vi "Teleop.vi"(10 "Match Info":T1={"Autonomous Elapsed Seconds"=0.0, "TeleOp Elapsed Seconds"=0.0, "Disabled Elapsed Seconds"=0.0, "Visited Autonomous"=FALSE, "Visited TeleOp"=FALSE, "Visited Disabled"=FALSE, "Autonomous Settings"={"Autonomous Style"=enum."Independent", "VI Refnum"=refnum}}, 11 "Call Context":T2) -> ()   [LabVIEW 2017]
doc: "This VI is called for each TeleOp packet received from the DS where the robot is not disabled. It is often used to read from the joysticks and update I/O or to update setpoints for timed control loops. It should complete and return within 20 milliseconds or it may miss DS packets."
uses:
  <vilib>/Rock Robotics/WPI/DriverStation/WPI_DriverStationDerivedRobotMode.ctl
  <vilib>/Rock Robotics/WPI/DriverStation/WPI_DriverStationMatch Info.ctl
  <vilib>/Rock Robotics/WPI/Solenoid/WPI_SolenoidValue.ctl
  <vilib>/Rock Robotics/WPI/Utilities/WPI_GetSetVariantRefNum.vi
  <vilib>/Rock Robotics/Network Tables/NT Write Numeric Array.vi
  <vilib>/Rock Robotics/Network Tables/NT Read Boolean.vi
  <vilib>/Rock Robotics/Network Tables/NT Read Number.vi
  <vilib>/Rock Robotics/Network Tables/NT Write Boolean Array.vi
  <vilib>/Rock Robotics/Network Tables/NT Write Number.vi
  <vilib>/Rock Robotics/WPI/Solenoid/WPI_SolenoidSetEnum.vi
panel:
  out "Sample Slider 0":dbl(slide) scale=0.0..5.0
  out "Sample Boolean 1":bool
  out "Sample Boolean 0":bool
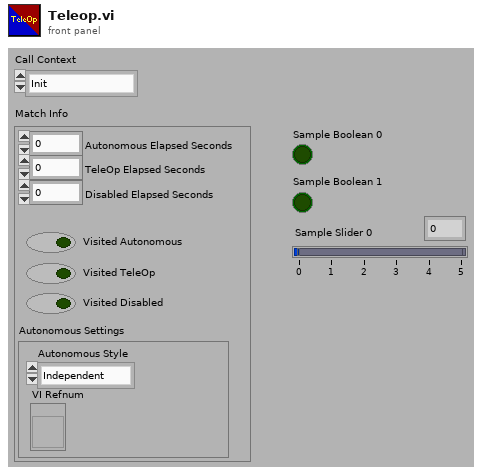
[diagram p1: front panel]
types:
  T1 = typedef "WPI_DriverStationMatch Info.ctl" = cluster{"Autonomous Elapsed Seconds":dbl, "TeleOp Elapsed Seconds":dbl, "Disabled Elapsed Seconds":dbl, "Visited Autonomous":bool, "Visited TeleOp":bool, "Visited Disabled":bool, "Autonomous Settings":cluster{"Autonomous Style":enum16{"Iterative", "Independent"}, "VI Refnum":refnum<vi>}}
  T2 = typedef "WPI_DriverStationDerivedRobotMode.ctl" = enum16{"Init", "Execute", "Stop"}
  T3 = typedef "WPI_SolenoidValue.ctl" = enum16{"Off", "On", "Forward", "Reverse"}
  T4 = typedef "WPI_JoystickDevRef.ctl" = cluster{"Device":T5}
  T5 = typedef "WPI_JoystickDeviceEnum.ctl" = enum16{"USB 0", "USB 1", "USB 2", "USB 3", "USB 4", "USB 5"}
  T6 = typedef "WPI_MotorControlDeviceRef.ctl" = cluster{"DeviceStatus":errorcluster, "Type":T7, "PWM":cluster{"PWM Channel":T8, "DeadBand":T9}, "CAN":cluster{"Device Number":u8, "SetOutput VI Ref":variant, "GetOutput VI Ref":variant, "Enable VI Ref":variant, "Disable VI Ref":variant, "Data":variant}, "Invert":bool, "DIO PWM":cluster{"PWM \"Enable\" Channel":T8, "DIOChannel":T10, "PWM Rate":dbl}}
  T7 = typedef "WPI_MotorControlType.ctl" = enum16{"PWM", "CAN", "DIO PWM"}
  T8 = typedef "FPGA_DIOPWMChannel.ctl" = enum8{"PWM 0", "PWM 1", "PWM 2", "PWM 3", "PWM 4", "PWM 5", "PWM 6", "PWM 7", "PWM 8", "PWM 9", "PWM MXP 0", "PWM MXP 1", "PWM MXP 2", "PWM MXP 3", "PWM MXP 4", "PWM MXP 5", "PWM MXP 6", "PWM MXP 7", "PWM MXP 8", "PWM MXP 9", "Invalid"}
  T9 = typedef "WPI_PWMDeadband.ctl" = cluster{"Name":string, "maxPositivePwm":i32, "minPositivePwm":i32, "centerPwm":i32, "maxNegativePwm":i32, "minNegativePwm":i32, "angularRange":u16}
  T10 = typedef "FPGA_DIOChannel.ctl" = enum8{"DIO 0", "DIO 1", "DIO 2", "DIO 3", "DIO 4", "DIO 5", "DIO 6", "DIO 7", "DIO 8", "DIO 9", "DIO MXP 0", "DIO MXP 1", "DIO MXP 2", "DIO MXP 3", "DIO MXP 4", "DIO MXP 5", "DIO MXP 6", "DIO MXP 7", "DIO MXP 8", "DIO MXP 9", "DIO MXP 10", "DIO MXP 11", "DIO MXP 12", "DIO MXP 13", "DIO MXP 14", "DIO MXP 15", "SPI Port CS1", "SPI Port CS2", "SPI Port CS3", "SPI Port MISO", "SPI Port MOSI", "Invalid"}
  T11 = typedef "WPI_SolenoidDevRef.ctl" = cluster{"DevStatus":errorcluster, "Pneumatics Control Module":u8, "Forward Solenoid Channel":T12, "Reverse Solenoid Channel":T12}
  T12 = typedef "WPI_SolenoidChannel.ctl" = enum8{"Solenoid 0", "Solenoid 1", "Solenoid 2", "Solenoid 3", "Solenoid 4", "Solenoid 5", "Solenoid 6", "Solenoid 7", "Invalid"}
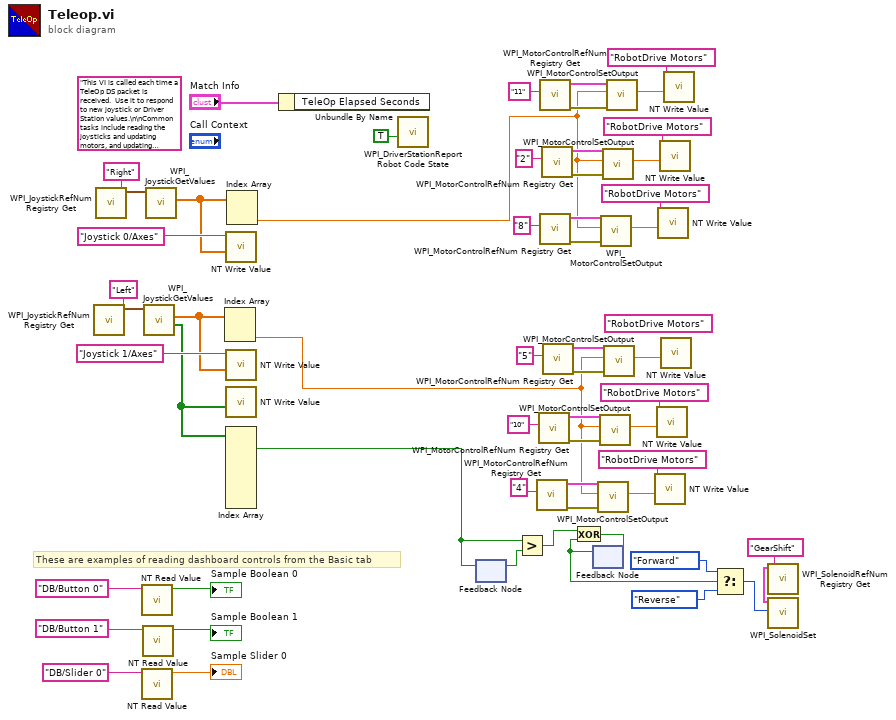
[diagram p0: block diagram]
diagram:
  (unwired) "RobotDrive Motors" ("Name")
  (unwired) "This VI is called each time a TeleOp DS packet is received.  Use it to respond to new joystick or Driver Station values.\n\nCommon tasks include reading the joysticks and updating motors, and updating setpoints for periodic loops.\n\nYou can open I/O on the FIRST Call, or in the Begin.vi."
  # "These are examples of reading dashboard controls from the Basic tab"
  n1 = call <vilib>:"WPI_JoystickRefNum Registry Get.vi"("refnum name"="Left") -> ("JoystickDevRef"=w44:T4)  [unwired: 1 in, 9 out]
  n2 = call <vilib>:"WPI_JoystickRefNum Registry Get.vi"("refnum name"="Right") -> ("JoystickDevRef"=w56:T4)  [unwired: 1 in, 9 out]
  n3 = call-poly <vilib>:"NT Read Value.vi"("Name"="DB/Button 0" ("refnum name")) -> ("Boolean"=→"Sample Boolean 0":bool)  [unwired: 9 in, 1 out]
  n4 = call-poly <vilib>:"NT Read Value.vi"("Name"="DB/Slider 0" ("refnum name")) -> ("Numeric"=→"Sample Slider 0":dbl)  [unwired: 9 in, 1 out]
  n5 = call-poly <vilib>:"NT Read Value.vi"("Name"="DB/Button 1" ("refnum name")) -> ("Boolean"=→"Sample Boolean 1":bool)  [unwired: 9 in, 1 out]
  n6 = call <vilib>:"WPI_JoystickGetValues.vi"("JoystickDevRef"=w44) -> ("Buttons"=w2:bool[], "Axes"=w42:dbl[])  [unwired: 6 in, 3 out]
  n7 = call <vilib>:"WPI_JoystickGetValues.vi"("JoystickDevRef"=w56) -> ("Axes"=w53:dbl[])  [unwired: 6 in, 4 out]
  n8 = Index Array(array=w42) -> (element #2=w13:dbl)  [unwired: 2 in, 1 out]
  n9 = call-poly <vilib>:"NT Write Value.vi"("Numeric Array"=w53, "Name"="Joystick 0/Axes") -> ()  [unwired: 9 in, 1 out]
  n10 = call-poly <vilib>:"NT Write Value.vi"("Numeric Array"=w42, "Name"="Joystick 1/Axes") -> ()  [unwired: 9 in, 1 out]
  n11 = call-poly <vilib>:"NT Write Value.vi"("Boolean Array"=w2) -> ()  [unwired: 10 in, 1 out]
  n12 = Index Array(array=w2) -> (element #1=w1:bool)  [unwired: 8 in, 7 out]
  n13 = Index Array(array=w53) -> (element #2=w12:dbl)  [unwired: 2 in, 1 out]
  n14 = Unbundle By Name("Match Info") -> ()  [unwired: 1 out]
  n15 = call <vilib>:"WPI_DriverStationReport Robot Code State.vi"("TeleOp"=TRUE ("Autonomous")) -> ()  [unwired: 10 in, 1 out]
  n16 = feedback #1() -> (w9:bool)  [unwired: 1 in]
  n17 = feedback-in #1(w1) -> ()
  n18 = Greater?(x=w1, y=w9) -> (0:w3:bool)
  n19 = call <vilib>:"WPI_MotorControlRefNum Registry Get.vi"("refnum name"="4") -> ("error out"=w22:errorcluster, "MotorControlDevRef"=w14:T6)  [unwired: 9 in]
  n20 = call <vilib>:"WPI_MotorControlRefNum Registry Get.vi"("refnum name"="10") -> ("error out"=w26:errorcluster, "MotorControlDevRef"=w15:T6)  [unwired: 9 in]
  n21 = call <vilib>:"WPI_MotorControlRefNum Registry Get.vi"("refnum name"="11") -> ("error out"=w41:errorcluster, "MotorControlDevRef"=w19:T6)  [unwired: 9 in]
  n22 = call <vilib>:"WPI_MotorControlRefNum Registry Get.vi"("refnum name"="8") -> ("error out"=w33:errorcluster, "MotorControlDevRef"=w18:T6)  [unwired: 9 in]
  n23 = call <vilib>:"WPI_MotorControlRefNum Registry Get.vi"("refnum name"="2") -> ("error out"=w37:errorcluster, "MotorControlDevRef"=w17:T6)  [unwired: 9 in]
  n24 = call <vilib>:"WPI_MotorControlRefNum Registry Get.vi"("refnum name"="5") -> ("error out"=w30:errorcluster, "MotorControlDevRef"=w16:T6)  [unwired: 9 in]
  n25 = feedback #2() -> (w10:bool)  [unwired: 1 in]
  n26 = Exclusive Or(1:w10, 2:w3) -> (0:w11:bool)
  n27 = feedback-in #2(w11) -> ()
  n28 = call <vilib>:"WPI_MotorControlSetOutput.vi"("error in (no error)"=w22, "Output"=w13, "MotorControlDevRef"=w14) -> ("Motor Output"=w20:dbl)  [unwired: 6 in, 2 out]
  n29 = call <vilib>:"WPI_MotorControlSetOutput.vi"("error in (no error)"=w26, "Output"=w13, "MotorControlDevRef"=w15) -> ("Motor Output"=w24:dbl)  [unwired: 6 in, 2 out]
  n30 = call <vilib>:"WPI_MotorControlSetOutput.vi"("error in (no error)"=w33, "Output"=w12, "MotorControlDevRef"=w18) -> ("Motor Output"=w31:dbl)  [unwired: 6 in, 2 out]
  n31 = call <vilib>:"WPI_MotorControlSetOutput.vi"("error in (no error)"=w37, "Output"=w12, "MotorControlDevRef"=w17) -> ("Motor Output"=w35:dbl)  [unwired: 6 in, 2 out]
  n32 = call <vilib>:"WPI_MotorControlSetOutput.vi"("error in (no error)"=w30, "Output"=w13, "MotorControlDevRef"=w16) -> ("Motor Output"=w28:dbl)  [unwired: 6 in, 2 out]
  n33 = call <vilib>:"WPI_MotorControlSetOutput.vi"("error in (no error)"=w41, "Output"=w12, "MotorControlDevRef"=w19) -> ("Motor Output"=w39:dbl)  [unwired: 6 in, 2 out]
  n34 = call-poly <vilib>:"NT Write Value.vi"("Numeric"=w20, "Name"="RobotDrive Motors") -> ()  [unwired: 9 in, 1 out]
  n35 = call-poly <vilib>:"NT Write Value.vi"("Numeric"=w24, "Name"="RobotDrive Motors") -> ()  [unwired: 9 in, 1 out]
  n36 = call-poly <vilib>:"NT Write Value.vi"("Numeric"=w31, "Name"="RobotDrive Motors") -> ()  [unwired: 9 in, 1 out]
  n37 = call-poly <vilib>:"NT Write Value.vi"("Numeric"=w35, "Name"="RobotDrive Motors") -> ()  [unwired: 9 in, 1 out]
  n38 = call-poly <vilib>:"NT Write Value.vi"("Numeric"=w28) -> ()  [unwired: 10 in, 1 out]
  n39 = call-poly <vilib>:"NT Write Value.vi"("Numeric"=w39, "Name"="RobotDrive Motors") -> ()  [unwired: 9 in, 1 out]
  n40 = Select(t=WPI_SolenoidValue."Forward" ("Value"), s=w10, f=WPI_SolenoidValue."Reverse" ("Value")) -> (s? t:f=w4:T3)
  n41 = call <vilib>:"WPI_SolenoidRefNum Registry Get.vi"("refnum name"="GearShift") -> ("SolenoidDevRef"=w7:T11)  [unwired: 9 in, 1 out]
  n42 = call-poly <vilib>:"WPI_SolenoidSet.vi"("Value"=w4, "SolenoidDevRef"=w7) -> ()  [unwired: 8 in, 2 out]
